vi "Retrieve and Dispatch Group.vi"(6 "command":T1, 7 "plugin iteration":u64=1, 8 "error in (no error)":errorcluster, 9 "plugin ID":i32, 10 "Dispatcher Interface in":refnum<class "Dispatcher Interface.lvclass">, 11 "Scheduler Transfer Group Bundle in":refnum<class "Scheduler Transfer Group Bundle.lvclass">) -> (0 "error out":errorcluster, 2 "Dispatcher Interface out":refnum<class "Dispatcher Interface.lvclass">, 3 "Scheduler Transfer Group Bundle out":refnum<class "Scheduler Transfer Group Bundle.lvclass">)   [LabVIEW 2017, in "DSF Core.lvlib" / "Scheduler Transfer Group Bundle.lvclass"]
uses:
  Scheduler Transfer Group Bundle.lvclass
  Interfaces/Dispatcher/Dispatcher Interface.lvclass
  Interfaces/Dispatcher/Command.ctl
  Scheduler Transfer Group Bundle.lvclass/Scheduler Transfer Group Bundle.ctl
  Timing/Timing.lvclass/Timing.ctl
  Timing/Get Decimation.vi
  Timing/Get Offset.vi
  Timing/Transfer Group Timing.lvclass
  C:/Git/DSF/Data Sharing Framework/Source/Core/Engine/Classes/Timing/Timing.lvclass
  Timing/Timing.lvclass
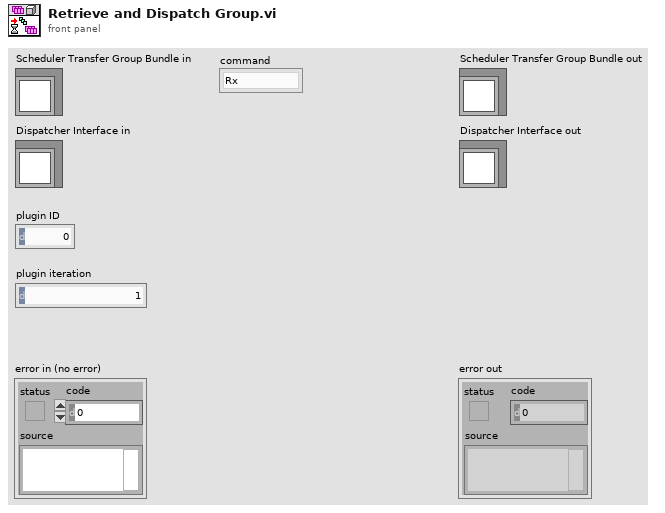
[diagram p1: front panel]
types:
  T1 = typedef "DSF Core.lvlib/Dispatcher Interface.lvclass/Command.ctl" = enum8{"Rx", "Tx", "Shutdown"}
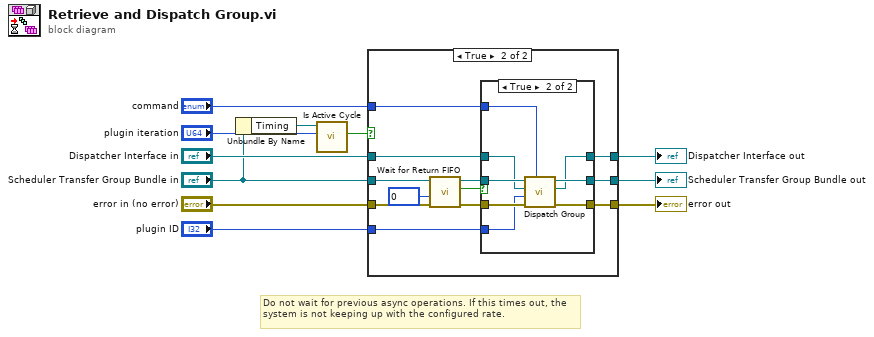
[diagram p0: block diagram]
diagram:
  # "Do not wait for previous async operations. If this times out, the system is not keeping up with the configured rate."
  n1 = Unbundle By Name("Scheduler Transfer Group Bundle in") -> ("Timing"=w4:refnum<class "Transfer Group Timing.lvclass">)
  n2 = call "Is Active Cycle.vi"("iteration"="plugin iteration", "Timing in"=w4) -> ("active?"=w5:bool)  [unwired: 8 in, 1 out]
  n3 = case shown="True" w5 {
    tunnel: [w14 w24] -> w6
    tunnel: "error in (no error)" -> [w14 w25]
    tunnel: "plugin ID" -> [_ w23]
    tunnel: [w12 w19] -> w2
    tunnel: "Dispatcher Interface in" -> [w13 w18]
    tunnel: [w13 w17] -> w8
    tunnel: "Scheduler Transfer Group Bundle in" -> [w12 w16]
    tunnel: "command" -> [_ w15]
    frame False {
    }
    frame True {
      n4 = call "Wait for Return FIFO.vi"("error in (no error)"=w25, "timeout (0 ms)"=0, "Transfer Group Bundle in"=w16) -> ("error out"=w26:errorcluster, "iteration valid"=w20:bool, "Transfer Group Bundle out"=w21:refnum<class "Scheduler Transfer Group Bundle.lvclass">)  [unwired: 6 in]
      n5 = case shown="True" w20 {
        tunnel: [w28 w34] -> w24
        tunnel: w23 -> [_ w31]
        tunnel: w26 -> [w28 w35]
        tunnel: w21 -> [w29 w37]
        tunnel: [w29 w36] -> w19
        tunnel: w18 -> [w27 w33]
        tunnel: [w27 w32] -> w17
        tunnel: w15 -> [_ w30]
        frame False {
        }
        frame True {
          n6 = call "Dispatch Group.vi"("command"=w30, "error in (no error)"=w35, "Plugin ID"=w31, "Dispatcher Interface in"=w33, "Scheduler Transfer Group Bundle in"=w37) -> ("error out"=w34:errorcluster, "Dispatcher Interface out"=w32:refnum<class "Dispatcher Interface.lvclass">, "Scheduler Transfer Group Bundle out"=w36:refnum<class "Scheduler Transfer Group Bundle.lvclass">)  [unwired: 4 in]
        }
      }
    }
  }
  "error out" <- w6
  "Scheduler Transfer Group Bundle out" <- w2
  "Dispatcher Interface out" <- w8
